vi "capstone1 ver 3.vi"() -> ()   [LabVIEW 2016]
uses:
  <instrlib>/Dynamixel Motor/Public/Motor Operation/Low Level/Baud Setting.ctl
  <vilib>/myRIO/Instrument Drivers/Onboard IO/DIO/typedefs/DIO Reference.ctl
  <vilib>/myRIO/Common/Instrument Driver Framework/Utilities/typedefs/myRIO Generic Hardware Reference.ctl
  <vilib>/myRIO/Common/Instrument Driver Framework/Utilities/typedefs/Hardware Version Enum.ctl
  <vilib>/myRIO/Common/Instrument Driver Framework/Utilities/typedefs/myRIO v1.0 Reference.ctl
  <vilib>/myRIO/Common/Instrument Driver Framework/Utilities/typedefs/Generic FPGA Reference.ctl
  <vilib>/myRIO/Common/Instrument Driver Framework/myRIO v1.0/DIO/typedefs/DIO Channels List.ctl
  <vilib>/myRIO/Common/Instrument Driver Framework/myRIO v1.0/DIO/typedefs/DIO Channels Enum.ctl
  <vilib>/userdefined/High Color/nirio_resource_hc.ctl
  <vilib>/myRIO/Common/Instrument Driver Framework/Utilities/vis/Is FPGA Ref Available.vi
  <vilib>/myRIO/Common/Instrument Driver Framework/myRIO v1.0/DIO/vis/myRIO v1.1 Open DIO.vi
  <vilib>/myRIO/Instrument Drivers/Onboard IO/DIO/vis/Write.vi
  <vilib>/myRIO/Common/Instrument Driver Framework/Utilities/vis/Validate Channels.vi
  <vilib>/myRIO/Common/Instrument Driver Framework/myRIO v1.0/DIO/vis/myRIO v1.0 Reserve DIO.vi
  <vilib>/myRIO/Common/Instrument Driver Framework/myRIO v1.0/Resource Manager/vis/myRIO v1.0 Reserve Channel List.vi
  <vilib>/myRIO/Common/Instrument Driver Framework/myRIO v1.0/DIO/vis/myRIO v1.0 Build MUX Configuration DIO.vi
  <vilib>/myRIO/Common/Instrument Driver Framework/myRIO v1.0/Resource Manager/vis/myRIO v1.0 Reserve Channel.vi
  <vilib>/myRIO/Common/Instrument Driver Framework/myRIO v1.0/Resource Manager/vis/myRIO v1.0 Unreserve Channel.vi
  <vilib>/myRIO/Common/Instrument Driver Framework/myRIO v1.0/Resource Manager/vis/myRIO v1.0 Create Configuration List.vi
  <vilib>/myRIO/Common/Instrument Driver Framework/myRIO v1.0/Resource Manager/vis/myRIO v1.0 Build Mutex Name.vi
  <vilib>/Utility/VariantDataType/GetNumericInfo.vi
  <vilib>/Utility/error.llb/Error Cluster From Error Code.vi
  <vilib>/myRIO/Common/Instrument Driver Framework/myRIO v1.0/myRIO v1.1 Open.vi
  <vilib>/myRIO/Common/Instrument Driver Framework/Utilities/vis/IO Manager.vi
  <vilib>/myRIO/Common/Instrument Driver Framework/Utilities/vis/Configuration Manager.vi
  <vilib>/myRIO/Common/Instrument Driver Framework/myRIO v1.0/Resource Manager/vis/myRIO v1.0 Configure IO.vi
  <vilib>/myRIO/Common/Instrument Driver Framework/myRIO v1.0/myRIO v1.0 Close.vi
  <vilib>/myRIO/Common/Instrument Driver Framework/myRIO v1.0/DIO/vis/myRIO v1.0 Write DIO.vi
  <vilib>/myRIO/Express VI/Onboard Devices/LED/LED Express VI.xnode
  <vilib>/myRIO/Instrument Drivers/Onboard IO/DIO/vis/myRIO DIO Open.xnode
  <instrlib>/Dynamixel Motor/Dynamixel Motor.lvlib
  <vilib>/myRIO/Instrument Drivers/Onboard IO/DIO/DIO.lvlib
panel:
  out "value":T1
  out "TCP Read data":string
  in  "정지":bool
  out "error out":errorcluster
  out "RT TCP Loop time":u32
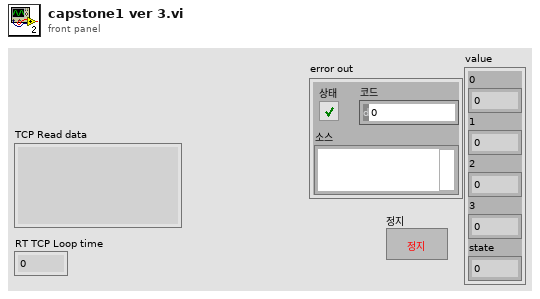
[diagram p1: front panel]
types:
  T1 = cluster{"0":sgl, "1":sgl, "2":sgl, "3":sgl, "state":sgl}
  T2 = typedef "Dynamixel Motor.lvlib/Baud Setting.ctl" = u8
  T3 = enum16{"big-endian, network order", "native, host order", "little-endian"}
  T4 = cluster{"0":sgl, "1":sgl, "2":sgl, "3":sgl, "state":i32}
  T5 = typedef "DIO.lvlib/DIO Reference.ctl" = cluster{"myRIO Reference":T6, "DIO Channels List":T10}
  T6 = typedef "myRIO Generic Hardware Reference.ctl" = cluster{"myRIO Model":T7, "myRIO Hardware Reference":T8}
  T7 = typedef "Hardware Version Enum.ctl" = enum16{"Unknown", "myRIO-1900", "myRIO-1950", "roboRIO", "NI ELVIS RIO CM"}
  T8 = typedef "myRIO v1.0 Reference.ctl" = cluster{"Generic FPGA Reference":T9, "Allow multiple opens":bool}
  T9 = typedef "Generic FPGA Reference.ctl" = refnum<k20>
  T10 = typedef "DIO Channels List.ctl" = T11[]
  T11 = typedef "DIO Channels Enum.ctl" = enum16{"Not Connected", "C/DIO0", "C/DIO1", "C/DIO2", "C/DIO3", "C/DIO4", "C/DIO5", "C/DIO6", "C/DIO7", "A/DIO0", "A/DIO1", "A/DIO2", "A/DIO3", "A/DIO4", "A/DIO5", "A/DIO6", "A/DIO7", "A/DIO8", "A/DIO9", "A/DIO10", "A/DIO11", "A/DIO12", "A/DIO13", "A/DIO14", "A/DIO15", "B/DIO0", "B/DIO1", "B/DIO2", "B/DIO3", "B/DIO4", "B/DIO5", "B/DIO6", "B/DIO7", "B/DIO8", "B/DIO9", "B/DIO10", "B/DIO11", "B/DIO12", "B/DIO13", "B/DIO14", "B/DIO15", "LED0", "LED1", "LED2", "LED3", "Button0", "DIO/DIO0", "DIO/DIO1", "DIO/DIO2", "DIO/DIO3", "DIO/DIO4", "DIO/DIO5", "DIO/DIO6", "DIO/DIO7", "DIO/DIO8", "DIO/DIO9", "SPI/CS0", "SPI/CS1", "SPI/CS2", "SPI/CS3", "LED RADIO (Green)", "LED RADIO (Red)", "LED COMM (Green)", "LED COMM (Red)", "LED MODE (Green)", "LED MODE (Red)"}
  T12 = typedef "nirio_resource_hc.ctl" = tag
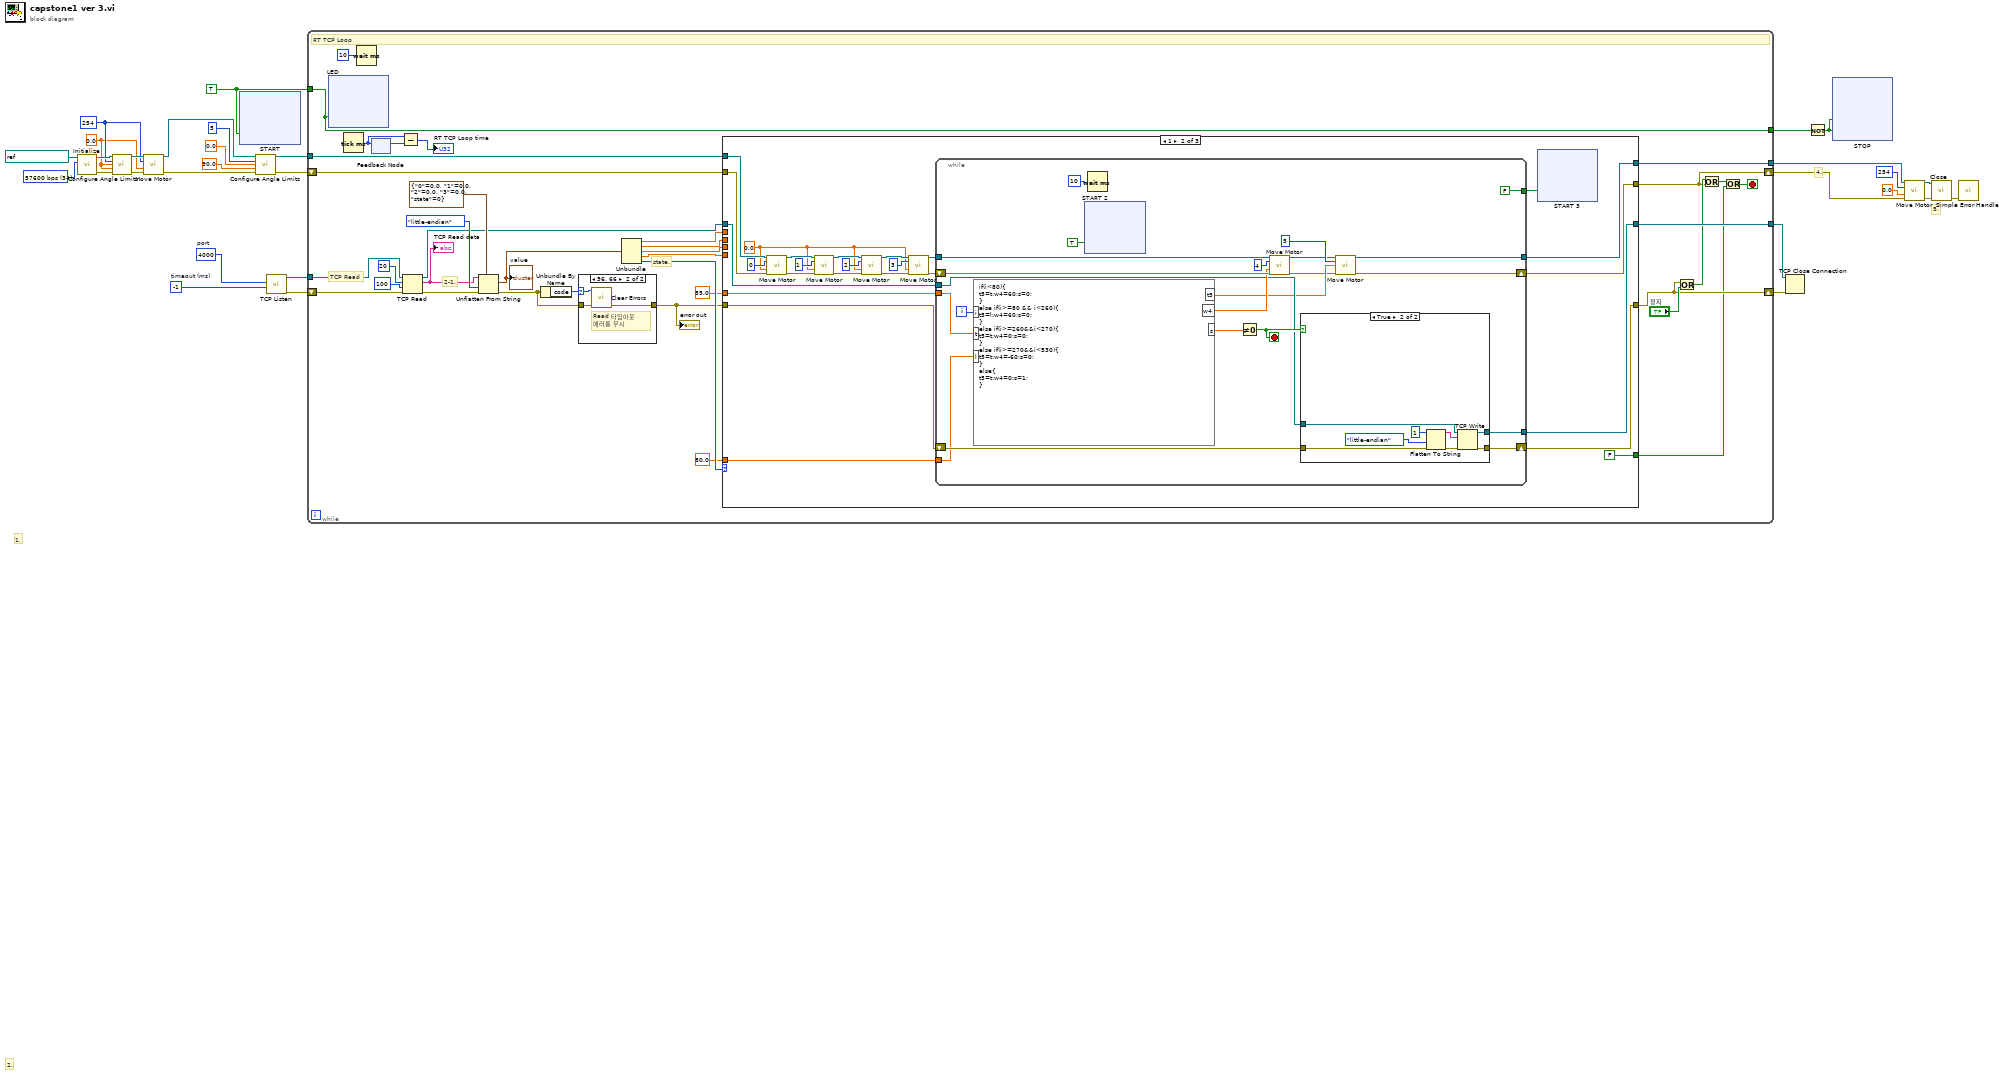
[diagram p0: block diagram]
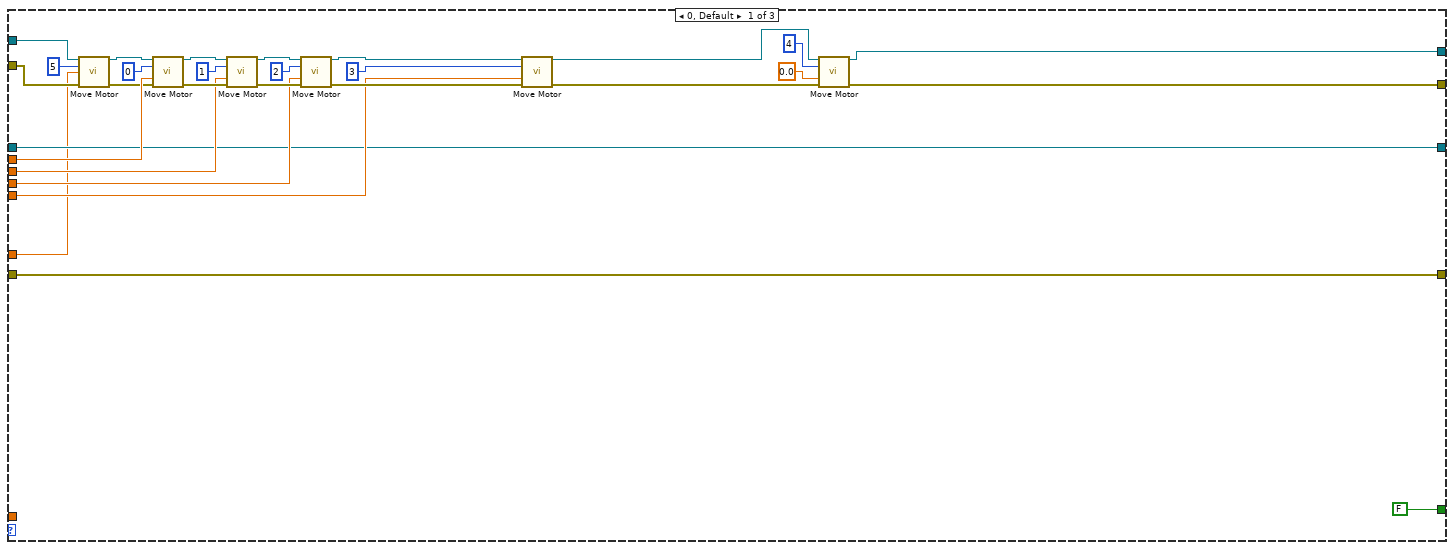
[diagram p2: hidden frame]
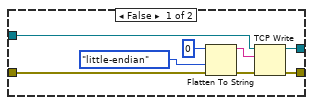
[diagram p3: hidden frame]
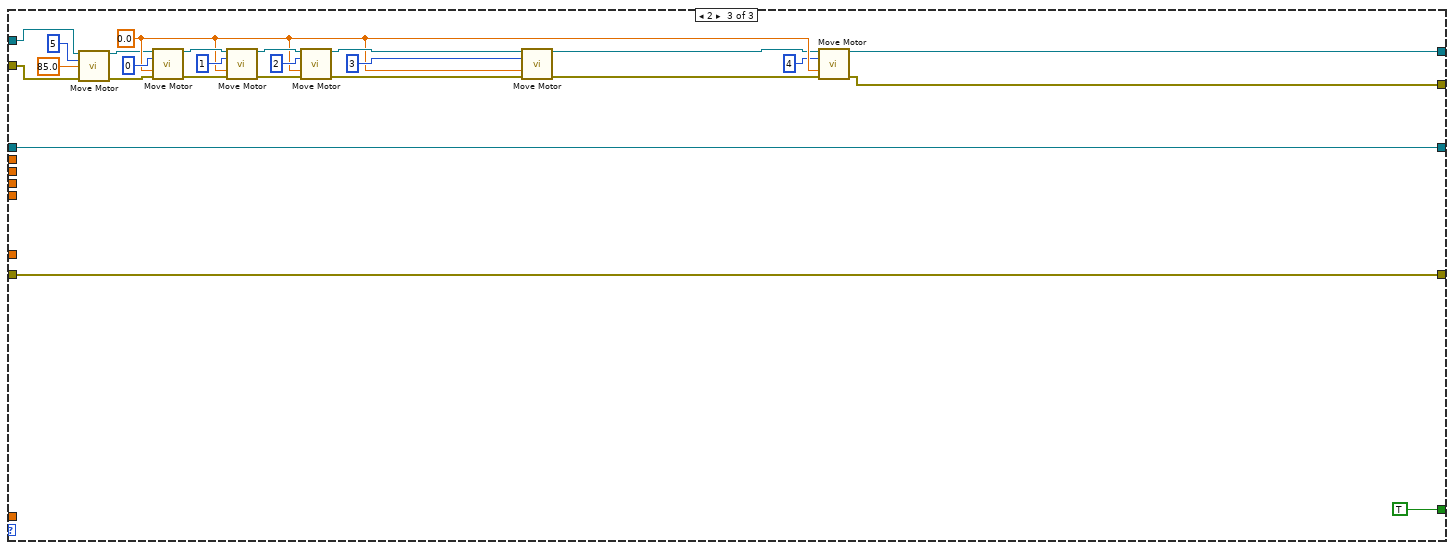
[diagram p4: hidden frame]
diagram:
  w25 = T2 34 items=["1,000,000 bps"=1, "500,000 bps"=3, "400,000 bps"=4, "250,000 bps"=7, "200,000 bps"=9, "115200 bps"=16, "57600 bps"=34, "19200 bps"=103, "9600 bps"=207] ("Baud rate (57600 bps)")
  w7 = TRUE
  w9 = u8 254 ("Motor ID (0)")
  w8 = 0.0 ("Clockwise Angle Limit (0 deg)")
  w30 = u16 4000  # port
  w31 = -1  # timeout (ms)
  # "5."
  # "4."
  # "2."
  # "1."
  n1 = call <instrlib>:"Initialize.vi"("Baud rate (57600 bps)"=w25, "VISA resource name"=refnum<visa-resource-name> "ASRL3::INSTR") -> ("error out"=w19:errorcluster, "VISA resource name out"=w18:refnum<visa-resource-name>)  [unwired: 8 in]
  n2 = call <instrlib>:"Configure Angle Limits.vi"("VISA resource name"=w18, "Motor ID (0)"=w9, "Clockwise Angle Limit (0 deg)"=w8, "Counter-Clockwise Angle Limit (300 deg)"=w8, "error in (no error)"=w19) -> ("VISA resource name out"=w11:refnum<visa-resource-name>, "error out"=w10:errorcluster)  [unwired: 9 in]
  n3 = call <instrlib>:"Move Motor.vi"("VISA resource name"=w11, "Motor ID (0)"=w9, "Goal Speed (RPM)"=w8, "error in (no error)"=w10) -> ("VISA resource name out"=w5:refnum<visa-resource-name>, "error out"=w6:errorcluster)  [unwired: 10 in]
  n4 = xnode "START"("LED0"=w7) -> ()  [unwired: 1 in, 1 out]
  n5 = call <instrlib>:"Configure Angle Limits.vi"("VISA resource name"=w5, "Motor ID (0)"=5, "Clockwise Angle Limit (0 deg)"=0.0, "Counter-Clockwise Angle Limit (300 deg)"=90.0 ("Clockwise Angle Limit (0 deg)"), "error in (no error)"=w6) -> ("VISA resource name out"=w15:refnum<visa-resource-name>, "error out"=w14:errorcluster)  [unwired: 9 in]
  n6 = call <vilib>:"TCP Listen.vi"("timeout ms (wait forever: -1)"=w31, "port"=w30) -> ("error out"=w26:errorcluster, "connection ID"=w27:refnum<k5>)  [unwired: 5 in, 3 out]
  n7 = while {
    tunnel: w27 -> [w53]
    tunnel: [w43] -> w29
    shift-right: [w38] -> w28
    shift-left: w26 -> [w54]
    shift-right: [w37] -> w4
    shift-left: w14 -> [w46]
    tunnel: w7 -> [w52]
    tunnel: [w52] -> w21
    tunnel: w15 -> [w41]
    tunnel: [w40] -> w3
    stop <- w32 stop-if-true
    # "state."
    # "2-1."
    # "TCP Read"
    # "RT TCP Loop"
    n8 = xnode "LED"("LED1"=w52) -> ()  [unwired: 1 in, 1 out]
    n9 = Tick Count (ms)() -> (millisecond timer value=w63:u32)
    n10 = Wait (ms)(milliseconds to wait=u32 10 ("대기 시간 (ms)")) -> ()  [unwired: 1 out]
    n11 = feedback #1() -> (w64:u32)  [unwired: 1 in]
    n12 = feedback-in #1(w63) -> ()
    n13 = Subtract(x=w63, y=w64) -> (x-y=→"RT TCP Loop time":u32)
    n14 = TCP Read(connection ID=w53, bytes to read=20 ("읽을 바이트"), error in (no error)=w54, 9:100 ("타임아웃 ms (25000)")) -> (connection ID out=w44:refnum<k5>, data out=w57:string, error out=w56:errorcluster)  [unwired: 1 in]
    "TCP Read data" <- w57
    n15 = Unflatten From String(type=T4 {"0"=0.0, "1"=0.0, "2"=0.0, "3"=0.0, "state"=0}, binary string=w57, byte order (0:big-endian, network order)=T3."little-endian", error in (no error)=w56) -> (value=w51:T4, error out=w55:errorcluster)  [unwired: 1 in, 1 out]
    "value" <- w51
    n16 = Unbundle By Name(w55) -> ("code"=w65:i32)
    n17 = case shown="56, 66" w65 {
      selector: w65 -> [_ w292]
      tunnel: [w290 w291] -> w42
      tunnel: w55 -> [w290 w293]
      frame 0, Default {
      }
      frame 56, 66 {
        # "Read 타임아웃\n에러를 무시"
        n18 = call <vilib>:"Clear Errors.vi"("error in (no error)"=w293, "specific error code to clear (0: all)"=w292) -> ("error out"=w291:errorcluster)  [unwired: 4 in, 1 out]
      }
    }
    "error out" <- w42
    n19 = Unbundle(w51) -> ("0"=w50:sgl, "1"=w48:sgl, "2"=w49:sgl, "3"=w47:sgl, "state"=w45:i32)
    n20 = case shown="1" w45 {
      tunnel: w50 -> [w86 _ _]
      tunnel: w48 -> [w85 _ _]
      tunnel: w49 -> [w84 _ _]
      tunnel: w47 -> [w83 _ _]
      tunnel: w41 -> [w71 w111 w233]
      tunnel: [w79 w106 w241] -> w40
      tunnel: [w77 w107 w240] -> w37
      tunnel: w46 -> [w81 w100 w237]
      tunnel: w44 -> [w74 w105 w236]
      tunnel: [w74 w102 w236] -> w43
      tunnel: w42 -> [w73 w104 w235]
      tunnel: [w73 w103 w235] -> w38
      tunnel: 55.0 -> [w69 w99 _]
      tunnel: 80.0 -> [_ w98 _]
      tunnel: [FALSE FALSE TRUE] -> w34
      frame 0, Default {
        n21 = call <instrlib>:"Move Motor.vi"("VISA resource name"=w71, "Motor ID (0)"=5, "Goal Position (180 deg)"=w69, "error in (no error)"=w81) -> ("VISA resource name out"=w70:refnum<visa-resource-name>, "error out"=w72:errorcluster)  [unwired: 10 in]
        n22 = call <instrlib>:"Move Motor.vi"("VISA resource name"=w70, "Motor ID (0)"=0, "Goal Speed (RPM)"=w86, "error in (no error)"=w72) -> ("VISA resource name out"=w87:refnum<visa-resource-name>, "error out"=w88:errorcluster)  [unwired: 10 in]
        n23 = call <instrlib>:"Move Motor.vi"("VISA resource name"=w87, "Motor ID (0)"=1, "Goal Speed (RPM)"=w85, "error in (no error)"=w88) -> ("VISA resource name out"=w89:refnum<visa-resource-name>, "error out"=w91:errorcluster)  [unwired: 10 in]
        n24 = call <instrlib>:"Move Motor.vi"("VISA resource name"=w89, "Motor ID (0)"=2, "Goal Speed (RPM)"=w84, "error in (no error)"=w91) -> ("VISA resource name out"=w90:refnum<visa-resource-name>, "error out"=w92:errorcluster)  [unwired: 10 in]
        n25 = call <instrlib>:"Move Motor.vi"("VISA resource name"=w90, "Motor ID (0)"=3, "Goal Speed (RPM)"=w83, "error in (no error)"=w92) -> ("VISA resource name out"=w80:refnum<visa-resource-name>, "error out"=w78:errorcluster)  [unwired: 10 in]
        n26 = call <instrlib>:"Move Motor.vi"("VISA resource name"=w80, "Motor ID (0)"=4, "Goal Speed (RPM)"=0.0, "error in (no error)"=w78) -> ("VISA resource name out"=w79:refnum<visa-resource-name>, "error out"=w77:errorcluster)  [unwired: 10 in]
      }
      frame 1 {
        w110 = 0.0
        n27 = call <instrlib>:"Move Motor.vi"("VISA resource name"=w111, "Motor ID (0)"=0, "Goal Speed (RPM)"=w110, "error in (no error)"=w100) -> ("VISA resource name out"=w112:refnum<visa-resource-name>, "error out"=w113:errorcluster)  [unwired: 10 in]
        n28 = call <instrlib>:"Move Motor.vi"("VISA resource name"=w112, "Motor ID (0)"=1, "Goal Speed (RPM)"=w110, "error in (no error)"=w113) -> ("VISA resource name out"=w114:refnum<visa-resource-name>, "error out"=w116:errorcluster)  [unwired: 10 in]
        n29 = call <instrlib>:"Move Motor.vi"("VISA resource name"=w114, "Motor ID (0)"=2, "Goal Speed (RPM)"=w110, "error in (no error)"=w116) -> ("VISA resource name out"=w115:refnum<visa-resource-name>, "error out"=w117:errorcluster)  [unwired: 10 in]
        n30 = call <instrlib>:"Move Motor.vi"("VISA resource name"=w115, "Motor ID (0)"=3, "Goal Speed (RPM)"=w110, "error in (no error)"=w117) -> ("VISA resource name out"=w108:refnum<visa-resource-name>, "error out"=w109:errorcluster)  [unwired: 10 in]
        n31 = while {
          shift-right: [w163] -> w107
          shift-left: w109 -> [w176]
          shift-right: [w168] -> w103
          shift-left: w104 -> [w169]
          tunnel: w105 -> [w170]
          tunnel: [w167] -> w102
          tunnel: [FALSE] -> w101
          tunnel: w108 -> [w177]
          tunnel: [w164] -> w106
          tunnel: w99 -> [w160]
          tunnel: w98 -> [w159]
          i -> [w174]
          stop <- w171 stop-if-true
          n32 = formula code="if(i<80){\nt5=t;w4=60;s=0;\n}\nelse if(i>=80 && i<260){\nt5=l;w4=60;s=0;\n}\nelse if(i>=260&&i<270){\nt5=t;w4=0;s=0;\n}\nelse if(i>=270&&i<530){\nt5=t;w4=-60;s=0;\n}\nelse{\nt5=t;w4=0;s=1;\n}"("i"=w174, "t"=w160, "l"=w159) -> ("t5"=w161:dbl, "w4"=w173:dbl, "s"=w172:dbl)
          n33 = xnode "START 2"("LED2"=TRUE) -> ()  [unwired: 1 in, 1 out]
          n34 = Wait (ms)(milliseconds to wait=u32 10 ("대기 시간 (ms)")) -> ()  [unwired: 1 out]
          n35 = Not Equal To 0?(x=w172) -> (x != 0?=w171:bool)
          n36 = call <instrlib>:"Move Motor.vi"("VISA resource name"=w177, "Motor ID (0)"=4, "Goal Speed (RPM)"=w173, "error in (no error)"=w176) -> ("VISA resource name out"=w158:refnum<visa-resource-name>, "error out"=w157:errorcluster)  [unwired: 10 in]
          n37 = case shown="True" w171 {
            tunnel: w170 -> [w217 w229]
            tunnel: [w215 w225] -> w167
            tunnel: w169 -> [w216 w224]
            tunnel: [w214 w222] -> w168
            frame False {
              n38 = Flatten To String(anything=0, byte order (0:big-endian, network order)=T3."little-endian", error in (no error)=w216) -> (data string=w219:string, error out=w218:errorcluster)  [unwired: 1 in, 1 out]
              n39 = TCP Write(connection ID=w217, data in=w219, error in (no error)=w218) -> (connection ID out=w215:refnum<k5>, error out=w214:errorcluster)  [unwired: 1 in, 1 out]
            }
            frame True {
              n40 = Flatten To String(anything=1, byte order (0:big-endian, network order)=T3."little-endian", error in (no error)=w224) -> (data string=w226:string, error out=w223:errorcluster)  [unwired: 1 in, 1 out]
              n41 = TCP Write(connection ID=w229, data in=w226, error in (no error)=w223) -> (connection ID out=w225:refnum<k5>, error out=w222:errorcluster)  [unwired: 1 in, 1 out]
            }
          }
          n42 = call <instrlib>:"Move Motor.vi"("VISA resource name"=w158, "Motor ID (0)"=5, "Goal Position (180 deg)"=w161, "error in (no error)"=w157) -> ("VISA resource name out"=w164:refnum<visa-resource-name>, "error out"=w163:errorcluster)  [unwired: 10 in]
        }
        n43 = xnode "START 3"("LED2"=w101) -> ()  [unwired: 1 in, 1 out]
      }
      frame 2 {
        w244 = 0.0
        n44 = call <instrlib>:"Move Motor.vi"("VISA resource name"=w233, "Motor ID (0)"=5, "Goal Position (180 deg)"=85.0, "error in (no error)"=w237) -> ("VISA resource name out"=w232:refnum<visa-resource-name>, "error out"=w234:errorcluster)  [unwired: 10 in]
        n45 = call <instrlib>:"Move Motor.vi"("VISA resource name"=w232, "Motor ID (0)"=0, "Goal Speed (RPM)"=w244, "error in (no error)"=w234) -> ("VISA resource name out"=w254:refnum<visa-resource-name>, "error out"=w253:errorcluster)  [unwired: 10 in]
        n46 = call <instrlib>:"Move Motor.vi"("VISA resource name"=w254, "Motor ID (0)"=1, "Goal Speed (RPM)"=w244, "error in (no error)"=w253) -> ("VISA resource name out"=w252:refnum<visa-resource-name>, "error out"=w250:errorcluster)  [unwired: 10 in]
        n47 = call <instrlib>:"Move Motor.vi"("VISA resource name"=w252, "Motor ID (0)"=2, "Goal Speed (RPM)"=w244, "error in (no error)"=w250) -> ("VISA resource name out"=w251:refnum<visa-resource-name>, "error out"=w249:errorcluster)  [unwired: 10 in]
        n48 = call <instrlib>:"Move Motor.vi"("VISA resource name"=w251, "Motor ID (0)"=3, "Goal Speed (RPM)"=w244, "error in (no error)"=w249) -> ("VISA resource name out"=w242:refnum<visa-resource-name>, "error out"=w239:errorcluster)  [unwired: 10 in]
        n49 = call <instrlib>:"Move Motor.vi"("VISA resource name"=w242, "Motor ID (0)"=4, "Goal Speed (RPM)"=w244, "error in (no error)"=w239) -> ("VISA resource name out"=w241:refnum<visa-resource-name>, "error out"=w240:errorcluster)  [unwired: 10 in]
      }
    }
    n50 = Or(x=w38, y="정지") -> (x .or. y?=w39:bool)
    n51 = Or(x=w39, y=w37) -> (x .or. y?=w33:bool)
    n52 = Or(x=w33, y=w34) -> (x .or. y?=w32:bool)
  }
  n53 = TCP Close Connection(connection ID=w29, error in (no error)=w28) -> ()  [unwired: 3 out]
  n54 = Not(x=w21) -> (.not. x?=w20:bool)
  n55 = xnode "STOP"("LED0"=w20, "LED1"=w20) -> ()  [unwired: 1 in, 1 out]
  n56 = call <instrlib>:"Move Motor.vi"("VISA resource name"=w3, "Motor ID (0)"=u8 254, "Goal Speed (RPM)"=0.0, "error in (no error)"=w4) -> ("VISA resource name out"=w2:refnum<visa-resource-name>, "error out"=w1:errorcluster)  [unwired: 10 in]
  n57 = call <instrlib>:"Close.vi"("error in (no error)"=w1, "VISA resource name"=w2) -> ("error out"=w13:errorcluster)  [unwired: 9 in]
  n58 = call <vilib>:"Simple Error Handler.vi"("error in (no error)"=w13) -> ()  [unwired: 4 in, 5 out]
